vi "ICG_WD.vi"() -> ()   [LabVIEW 2020]
uses:
  <vilib>/Utility/file.llb/Read Delimited Spreadsheet (DBL).vi
  <vilib>/Analysis/NI_AALPro.lvlib
panel:
  out "SV 4":dbl
  out "SV 3":dbl
  out "SV 2":dbl
  out "SV":dbl
  out "SV":dbl
  out "Tlve 5":dbl
  out "interval7 2":dbl[](graph)
  out "location 5":dbl[](array[numeric])
  out "interval 7":dbl[](array[numeric])
  out "amplitude 5":dbl[](array[numeric])
  out "Amplitudes 5":dbl[](array[numeric])
  out "2nd Derivatives 5":dbl[](array[numeric])
  out "Locations 5":dbl[](array[numeric])
  out "max  4":dbl
  out "deltaZe(t)4 2":dbl[](graph)
  out "ICG array 5":dbl[](array[numeric])
  in  "file path (dialog if empty) 5":path
  out "Tlve 4":dbl
  out "interval7":dbl[](graph)
  out "location 4":dbl[](array[numeric])
  out "interval 6":dbl[](array[numeric])
  out "amplitude 4":dbl[](array[numeric])
  out "Amplitudes 4":dbl[](array[numeric])
  out "2nd Derivatives 4":dbl[](array[numeric])
  out "Locations 4":dbl[](array[numeric])
  out "max  3":dbl
  out "deltaZe(t)4":dbl[](graph)
  out "ICG array 4":dbl[](array[numeric])
  in  "file path (dialog if empty) 4":path
  out "Tlve 3":dbl
  out "interval 5":dbl[](graph)
  out "location 3":dbl[](array[numeric])
  out "interval 4":dbl[](array[numeric])
  out "amplitude 3":dbl[](array[numeric])
  out "Amplitudes 3":dbl[](array[numeric])
  out "2nd Derivatives 3":dbl[](array[numeric])
  out "Locations 3":dbl[](array[numeric])
  out "max  2":dbl
  out "deltaZe(t) 3":dbl[](graph)
  out "ICG array 3":dbl[](array[numeric])
  in  "file path (dialog if empty) 3":path
  out "Tlve 2":dbl
  out "interval 3":dbl[](graph)
  out "location 2":dbl[](array[numeric])
  out "interval 2":dbl[](array[numeric])
  out "amplitude 2":dbl[](array[numeric])
  out "Amplitudes 2":dbl[](array[numeric])
  out "2nd Derivatives 2":dbl[](array[numeric])
  out "Locations 2":dbl[](array[numeric])
  out "max  2":dbl
  out "deltaZe(t) 2":dbl[](graph)
  out "ICG":dbl[](array[numeric])
  in  "file path (dialog if empty) 2":path
  out "Tlve":dbl
  out "interval":dbl[](graph)
  out "location":dbl[](array[numeric])
  out "interval":dbl[](array[numeric])
  out "amplitude":dbl[](array[numeric])
  out "Amplitudes":dbl[](array[numeric])
  out "2nd Derivatives":dbl[](array[numeric])
  out "Locations":dbl[](array[numeric])
  out "max":dbl
  out "deltaZe(t)":dbl[](graph)
  out "ICG":dbl[](array[numeric])
  in  "file path (dialog if empty)":path
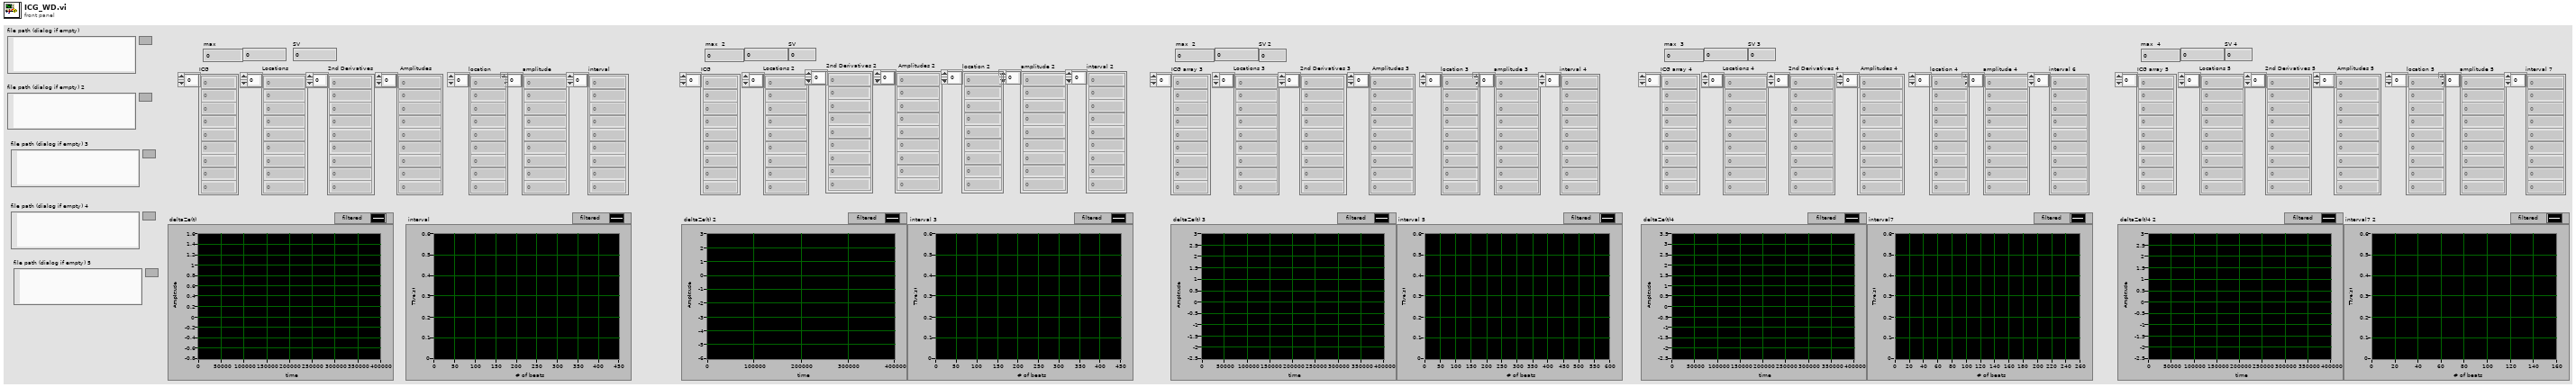
[diagram p1: front panel]
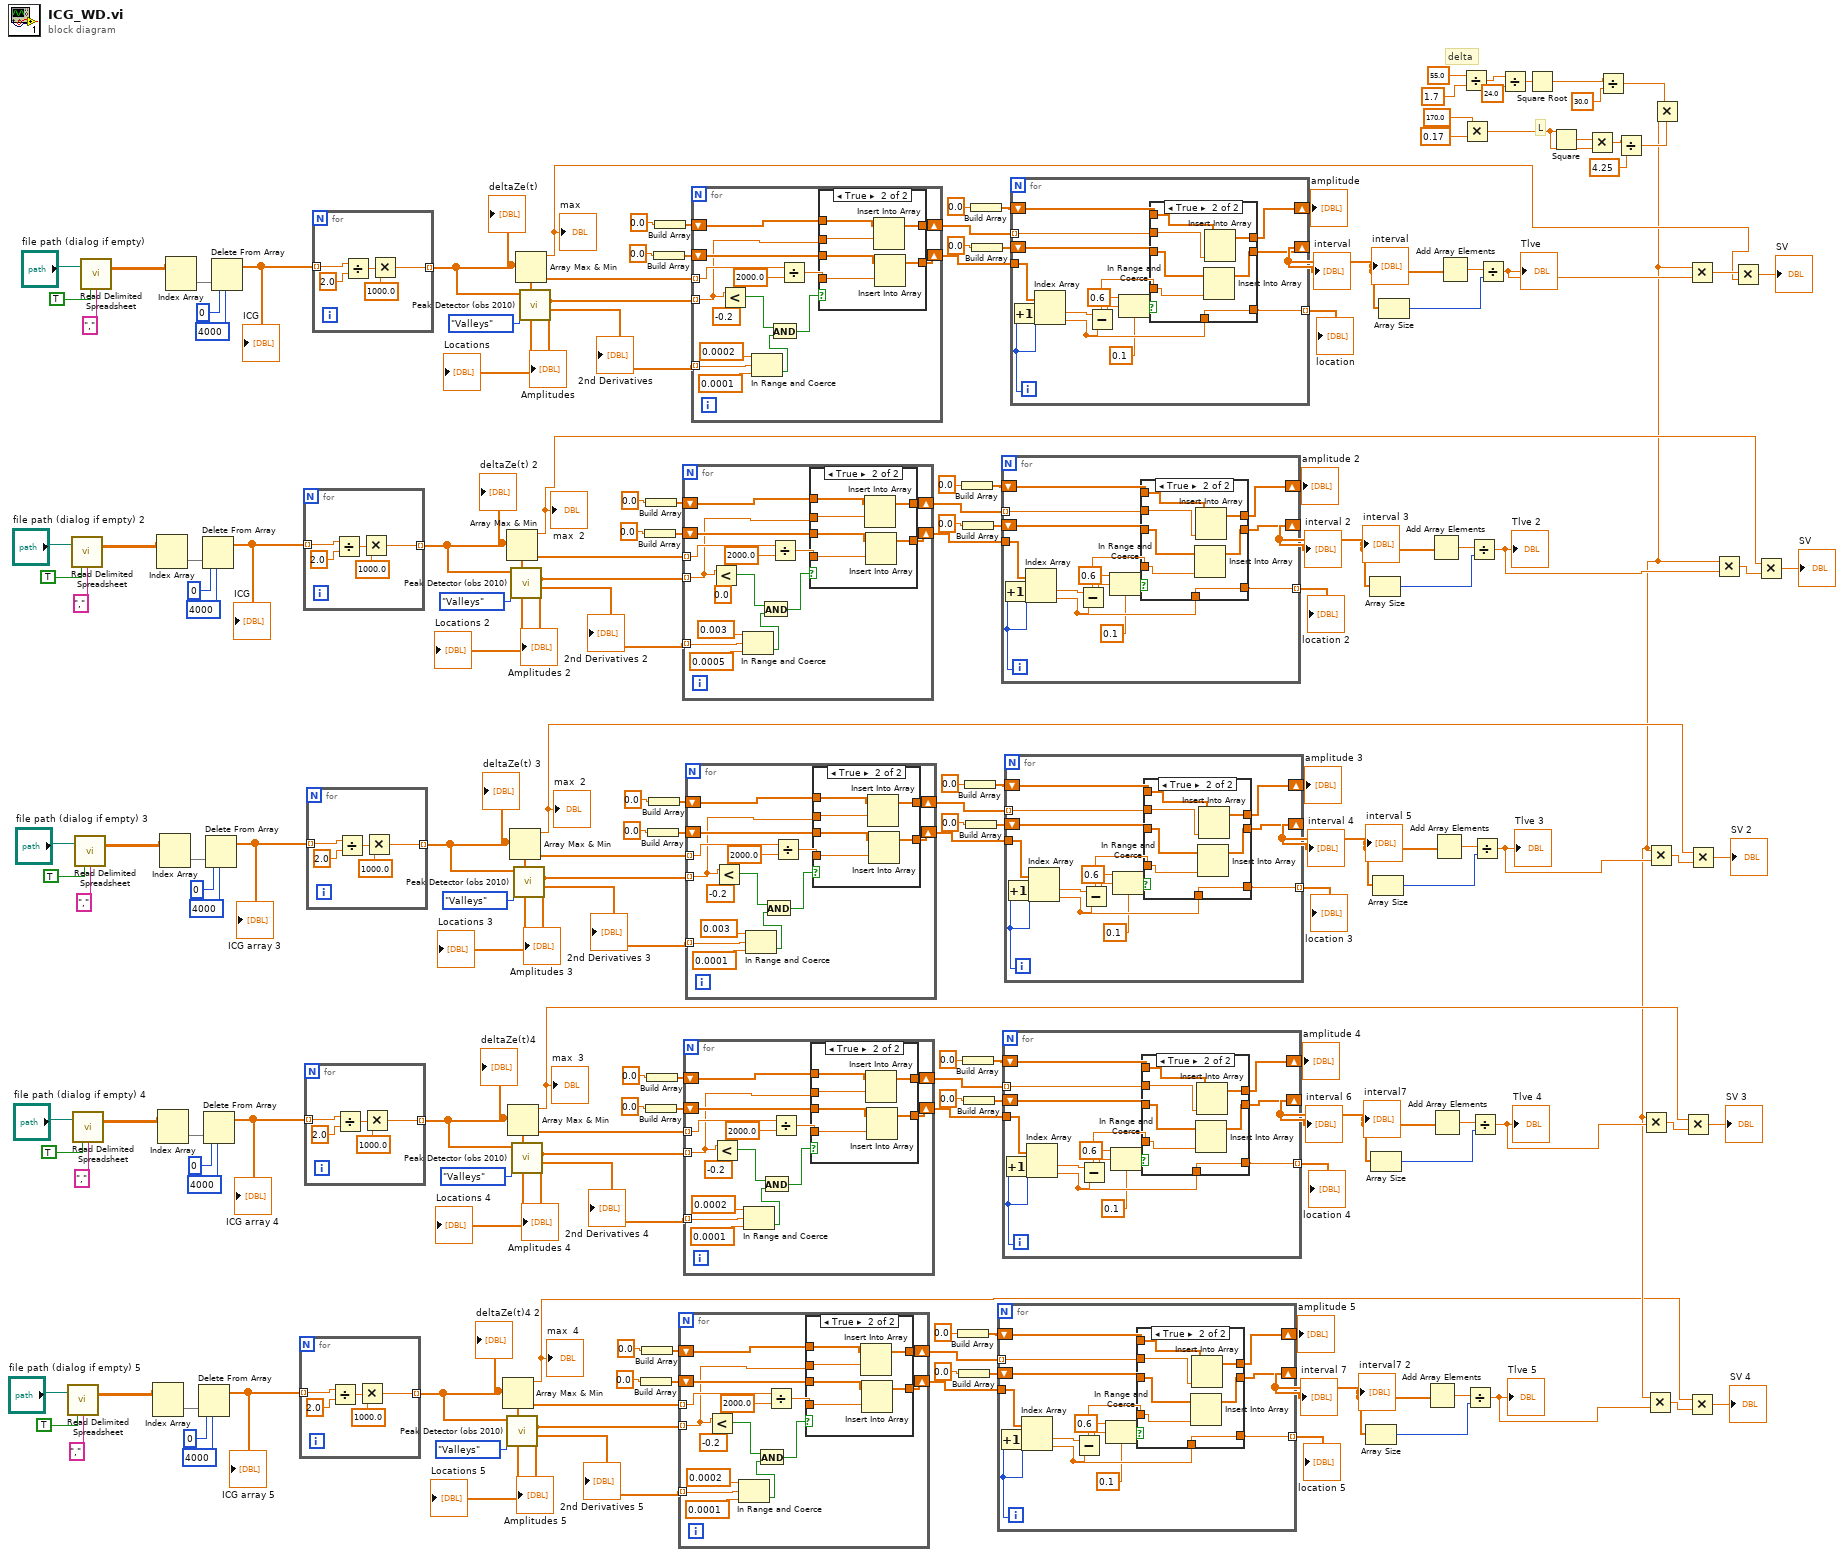
[diagram p0: block diagram]
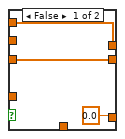
[diagram p2: hidden frame]
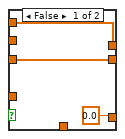
[diagram p4: hidden frame]
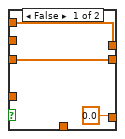
[diagram p6: hidden frame]
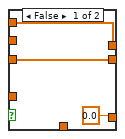
[diagram p8: hidden frame]
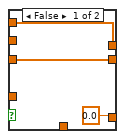
[diagram p10: hidden frame]
diagram:
  # "L"
  # "delta"
  n1 = call-poly <vilib>:"Read Delimited Spreadsheet.vi"("file path (dialog if empty)"="file path (dialog if empty) 5", "transpose? (F)"=TRUE, "delimiter (\\t)"="," ("delimiter (\\t)")) -> ("all rows"=w61:dbl[][])  [unwired: 7 in, 5 out]
  n2 = call-poly <vilib>:"Read Delimited Spreadsheet.vi"("file path (dialog if empty)"="file path (dialog if empty) 2", "transpose? (F)"=TRUE, "delimiter (\\t)"="," ("delimiter (\\t)")) -> ("all rows"=w145:dbl[][])  [unwired: 7 in, 5 out]
  n3 = call-poly <vilib>:"Read Delimited Spreadsheet.vi"("file path (dialog if empty)"="file path (dialog if empty) 4", "transpose? (F)"=TRUE, "delimiter (\\t)"="," ("delimiter (\\t)")) -> ("all rows"=w89:dbl[][])  [unwired: 7 in, 5 out]
  n4 = call-poly <vilib>:"Read Delimited Spreadsheet.vi"("file path (dialog if empty)"="file path (dialog if empty) 3", "transpose? (F)"=TRUE, "delimiter (\\t)"="," ("delimiter (\\t)")) -> ("all rows"=w117:dbl[][])  [unwired: 7 in, 5 out]
  n5 = call-poly <vilib>:"Read Delimited Spreadsheet.vi"("file path (dialog if empty)"="file path (dialog if empty)", "transpose? (F)"=TRUE, "delimiter (\\t)"="," ("delimiter (\\t)")) -> ("all rows"=w173:dbl[][])  [unwired: 7 in, 5 out]
  n6 = Index Array(array=w61) -> (element=w60:dbl[])  [unwired: 2 in]
  n7 = Index Array(array=w145) -> (element=w144:dbl[])  [unwired: 2 in]
  n8 = Index Array(array=w89) -> (element=w88:dbl[])  [unwired: 2 in]
  n9 = Index Array(array=w117) -> (element=w116:dbl[])  [unwired: 2 in]
  n10 = Index Array(array=w173) -> (element=w172:dbl[])  [unwired: 2 in]
  n11 = Delete From Array(array=w60, length=4000, index=0) -> (array with subset deleted=w57:dbl[])  [unwired: 1 out]
  "ICG array 5" <- w57
  n12 = Delete From Array(array=w144, length=4000, index=0) -> (array with subset deleted=w141:dbl[])  [unwired: 1 out]
  "ICG" <- w141
  n13 = Delete From Array(array=w88, length=4000, index=0) -> (array with subset deleted=w85:dbl[])  [unwired: 1 out]
  "ICG array 4" <- w85
  n14 = Delete From Array(array=w116, length=4000, index=0) -> (array with subset deleted=w113:dbl[])  [unwired: 1 out]
  "ICG array 3" <- w113
  n15 = Delete From Array(array=w172, length=4000, index=0) -> (array with subset deleted=w169:dbl[])  [unwired: 1 out]
  "ICG" <- w169
  n16 = for {
    tunnel: w57 -> [w181] mode=indexing
    tunnel: [w177] -> w53 mode=indexing
    n17 = Divide(x=w181, y=2.0) -> (x/y=w179:dbl)
    n18 = Multiply(x=w179, y=1000.0) -> (x*y=w177:dbl)
  }
  "deltaZe(t)4 2" <- w53
  n19 = for {
    tunnel: w141 -> [w186] mode=indexing
    tunnel: [w182] -> w137 mode=indexing
    n20 = Divide(x=w186, y=2.0) -> (x/y=w184:dbl)
    n21 = Multiply(x=w184, y=1000.0) -> (x*y=w182:dbl)
  }
  "deltaZe(t) 2" <- w137
  n22 = for {
    tunnel: w85 -> [w191] mode=indexing
    tunnel: [w187] -> w81 mode=indexing
    n23 = Divide(x=w191, y=2.0) -> (x/y=w189:dbl)
    n24 = Multiply(x=w189, y=1000.0) -> (x*y=w187:dbl)
  }
  "deltaZe(t)4" <- w81
  n25 = for {
    tunnel: w113 -> [w196] mode=indexing
    tunnel: [w192] -> w109 mode=indexing
    n26 = Divide(x=w196, y=2.0) -> (x/y=w194:dbl)
    n27 = Multiply(x=w194, y=1000.0) -> (x*y=w192:dbl)
  }
  "deltaZe(t) 3" <- w109
  n28 = for {
    tunnel: w169 -> [w201] mode=indexing
    tunnel: [w197] -> w165 mode=indexing
    n29 = Divide(x=w201, y=2.0) -> (x/y=w199:dbl)
    n30 = Multiply(x=w199, y=1000.0) -> (x*y=w197:dbl)
  }
  "deltaZe(t)" <- w165
  n31 = Array Max & Min(array=w53) -> (max value=w1:dbl)  [unwired: 3 out]
  "max  4" <- w1
  n32 = Array Max & Min(array=w137) -> (max value=w16:dbl)  [unwired: 3 out]
  "max  2" <- w16
  n33 = call <vilib>:"Peak Detector (obs 2010).vi"("peaks/valleys"=enum32{"Peaks", "Valleys"}."Valleys", "X"=w53) -> ("2nd Derivatives"=w51:dbl[], "Amplitudes"=w52:dbl[], "Locations"=w48:dbl[])  [unwired: 5 in, 2 out]
  "Locations 5" <- w48
  "2nd Derivatives 5" <- w51
  "Amplitudes 5" <- w52
  n34 = Array Max & Min(array=w81) -> (max value=w6:dbl)  [unwired: 3 out]
  "max  3" <- w6
  n35 = Array Max & Min(array=w109) -> (max value=w10:dbl)  [unwired: 3 out]
  "max  2" <- w10
  n36 = call <vilib>:"Peak Detector (obs 2010).vi"("peaks/valleys"=enum32{"Peaks", "Valleys"}."Valleys", "X"=w137) -> ("2nd Derivatives"=w135:dbl[], "Amplitudes"=w136:dbl[], "Locations"=w132:dbl[])  [unwired: 5 in, 2 out]
  "Locations 2" <- w132
  "2nd Derivatives 2" <- w135
  "Amplitudes 2" <- w136
  n37 = call <vilib>:"Peak Detector (obs 2010).vi"("peaks/valleys"=enum32{"Peaks", "Valleys"}."Valleys", "X"=w81) -> ("2nd Derivatives"=w79:dbl[], "Amplitudes"=w80:dbl[], "Locations"=w76:dbl[])  [unwired: 5 in, 2 out]
  "Locations 4" <- w76
  "2nd Derivatives 4" <- w79
  "Amplitudes 4" <- w80
  n38 = call <vilib>:"Peak Detector (obs 2010).vi"("peaks/valleys"=enum32{"Peaks", "Valleys"}."Valleys", "X"=w109) -> ("2nd Derivatives"=w107:dbl[], "Amplitudes"=w108:dbl[], "Locations"=w104:dbl[])  [unwired: 5 in, 2 out]
  "Locations 3" <- w104
  "2nd Derivatives 3" <- w107
  "Amplitudes 3" <- w108
  n39 = Array Max & Min(array=w165) -> (max value=w18:dbl)  [unwired: 3 out]
  "max" <- w18
  n40 = call <vilib>:"Peak Detector (obs 2010).vi"("peaks/valleys"=enum32{"Peaks", "Valleys"}."Valleys", "X"=w165) -> ("2nd Derivatives"=w163:dbl[], "Amplitudes"=w164:dbl[], "Locations"=w160:dbl[])  [unwired: 5 in, 2 out]
  "Locations" <- w160
  "2nd Derivatives" <- w163
  "Amplitudes" <- w164
  n41 = Build Array(0.0 ("array")) -> (w49:dbl[])
  n42 = Build Array(0.0 ("array")) -> (w54:dbl[])
  n43 = Build Array(0.0 ("array")) -> (w133:dbl[])
  n44 = Build Array(0.0 ("array")) -> (w138:dbl[])
  n45 = Build Array(0.0 ("array")) -> (w77:dbl[])
  n46 = Build Array(0.0 ("array")) -> (w82:dbl[])
  n47 = Build Array(0.0 ("array")) -> (w105:dbl[])
  n48 = Build Array(0.0 ("array")) -> (w110:dbl[])
  n49 = Build Array(0.0 ("array")) -> (w161:dbl[])
  n50 = Build Array(0.0 ("array")) -> (w166:dbl[])
  n51 = for {
    tunnel: w52 -> [w202] mode=indexing
    shift-right: [w214] -> w47
    shift-left: w54 -> [w215]
    tunnel: w51 -> [w209] mode=indexing
    shift-right: [w207] -> w46
    shift-left: w49 -> [w208]
    tunnel: w48 -> [w205] mode=indexing
    n52 = Less?(x=w202, y=-0.2) -> (x < y?=w211:bool)
    n53 = In Range and Coerce(upper limit=0.0002, x=w209, lower limit=0.0001) -> (In Range?=w206:bool)  [unwired: 1 out]
    n54 = And(x=w211, y=w206) -> (x .and. y?=w210:bool)
    n55 = Divide(x=w205, y=2000.0) -> (x/y=w203:dbl)
    n56 = case shown="True" w210 {
      tunnel: w215 -> [w218 w224]
      tunnel: [w218 w223] -> w214
      tunnel: w202 -> [_ w222]
      tunnel: w208 -> [w217 w221]
      tunnel: [w217 w220] -> w207
      tunnel: w203 -> [_ w219]
      frame False {
      }
      frame True {
        n57 = Insert Into Array(array=w224, new element=w222) -> (w223:dbl[])  [unwired: 1 in]
        n58 = Insert Into Array(array=w221, new element=w219) -> (w220:dbl[])  [unwired: 1 in]
      }
    }
  }
  n59 = for {
    tunnel: w136 -> [w225] mode=indexing
    shift-right: [w237] -> w131
    shift-left: w138 -> [w238]
    tunnel: w135 -> [w232] mode=indexing
    shift-right: [w230] -> w130
    shift-left: w133 -> [w231]
    tunnel: w132 -> [w228] mode=indexing
    n60 = Less?(x=w225, y=0.0) -> (x < y?=w234:bool)
    n61 = In Range and Coerce(upper limit=0.003, x=w232, lower limit=0.0005) -> (In Range?=w229:bool)  [unwired: 1 out]
    n62 = And(x=w234, y=w229) -> (x .and. y?=w233:bool)
    n63 = Divide(x=w228, y=2000.0) -> (x/y=w226:dbl)
    n64 = case shown="True" w233 {
      tunnel: w238 -> [w241 w247]
      tunnel: [w241 w246] -> w237
      tunnel: w225 -> [_ w245]
      tunnel: w231 -> [w240 w244]
      tunnel: [w240 w243] -> w230
      tunnel: w226 -> [_ w242]
      frame False {
      }
      frame True {
        n65 = Insert Into Array(array=w247, new element=w245) -> (w246:dbl[])  [unwired: 1 in]
        n66 = Insert Into Array(array=w244, new element=w242) -> (w243:dbl[])  [unwired: 1 in]
      }
    }
  }
  n67 = for {
    tunnel: w80 -> [w248] mode=indexing
    shift-right: [w260] -> w75
    shift-left: w82 -> [w261]
    tunnel: w79 -> [w255] mode=indexing
    shift-right: [w253] -> w74
    shift-left: w77 -> [w254]
    tunnel: w76 -> [w251] mode=indexing
    n68 = Less?(x=w248, y=-0.2) -> (x < y?=w257:bool)
    n69 = In Range and Coerce(upper limit=0.0002, x=w255, lower limit=0.0001) -> (In Range?=w252:bool)  [unwired: 1 out]
    n70 = And(x=w257, y=w252) -> (x .and. y?=w256:bool)
    n71 = Divide(x=w251, y=2000.0) -> (x/y=w249:dbl)
    n72 = case shown="True" w256 {
      tunnel: w261 -> [w264 w270]
      tunnel: [w264 w269] -> w260
      tunnel: w248 -> [_ w268]
      tunnel: w254 -> [w263 w267]
      tunnel: [w263 w266] -> w253
      tunnel: w249 -> [_ w265]
      frame False {
      }
      frame True {
        n73 = Insert Into Array(array=w270, new element=w268) -> (w269:dbl[])  [unwired: 1 in]
        n74 = Insert Into Array(array=w267, new element=w265) -> (w266:dbl[])  [unwired: 1 in]
      }
    }
  }
  n75 = for {
    tunnel: w108 -> [w271] mode=indexing
    shift-right: [w283] -> w103
    shift-left: w110 -> [w284]
    tunnel: w107 -> [w278] mode=indexing
    shift-right: [w276] -> w102
    shift-left: w105 -> [w277]
    tunnel: w104 -> [w274] mode=indexing
    n76 = Less?(x=w271, y=-0.2) -> (x < y?=w280:bool)
    n77 = In Range and Coerce(upper limit=0.003, x=w278, lower limit=0.0001) -> (In Range?=w275:bool)  [unwired: 1 out]
    n78 = And(x=w280, y=w275) -> (x .and. y?=w279:bool)
    n79 = Divide(x=w274, y=2000.0) -> (x/y=w272:dbl)
    n80 = case shown="True" w279 {
      tunnel: w284 -> [w287 w293]
      tunnel: [w287 w292] -> w283
      tunnel: w271 -> [_ w291]
      tunnel: w277 -> [w286 w290]
      tunnel: [w286 w289] -> w276
      tunnel: w272 -> [_ w288]
      frame False {
      }
      frame True {
        n81 = Insert Into Array(array=w293, new element=w291) -> (w292:dbl[])  [unwired: 1 in]
        n82 = Insert Into Array(array=w290, new element=w288) -> (w289:dbl[])  [unwired: 1 in]
      }
    }
  }
  n83 = for {
    tunnel: w164 -> [w294] mode=indexing
    shift-right: [w306] -> w159
    shift-left: w166 -> [w307]
    tunnel: w163 -> [w301] mode=indexing
    shift-right: [w299] -> w158
    shift-left: w161 -> [w300]
    tunnel: w160 -> [w297] mode=indexing
    n84 = Less?(x=w294, y=-0.2) -> (x < y?=w303:bool)
    n85 = In Range and Coerce(upper limit=0.0002, x=w301, lower limit=0.0001) -> (In Range?=w298:bool)  [unwired: 1 out]
    n86 = And(x=w303, y=w298) -> (x .and. y?=w302:bool)
    n87 = Divide(x=w297, y=2000.0) -> (x/y=w295:dbl)
    n88 = case shown="True" w302 {
      tunnel: w307 -> [w310 w316]
      tunnel: [w310 w315] -> w306
      tunnel: w294 -> [_ w314]
      tunnel: w300 -> [w309 w313]
      tunnel: [w309 w312] -> w299
      tunnel: w295 -> [_ w311]
      frame False {
      }
      frame True {
        n89 = Insert Into Array(array=w316, new element=w314) -> (w315:dbl[])  [unwired: 1 in]
        n90 = Insert Into Array(array=w313, new element=w311) -> (w312:dbl[])  [unwired: 1 in]
      }
    }
  }
  n91 = Build Array(0.0 ("array")) -> (w43:dbl[])
  n92 = Build Array(0.0 ("array")) -> (w44:dbl[])
  n93 = Build Array(0.0 ("array")) -> (w127:dbl[])
  n94 = Build Array(0.0 ("array")) -> (w128:dbl[])
  n95 = Build Array(0.0 ("array")) -> (w71:dbl[])
  n96 = Build Array(0.0 ("array")) -> (w72:dbl[])
  n97 = Build Array(0.0 ("array")) -> (w99:dbl[])
  n98 = Build Array(0.0 ("array")) -> (w100:dbl[])
  n99 = Build Array(0.0 ("array")) -> (w155:dbl[])
  n100 = Build Array(0.0 ("array")) -> (w156:dbl[])
  n101 = for {
    tunnel: w46 -> [w329]
    shift-right: [w325] -> w39
    shift-left: w44 -> [w326]
    tunnel: w47 -> [w321] mode=indexing
    shift-right: [w331] -> w41
    shift-left: w43 -> [w324]
    tunnel: [w322] -> w40 mode=indexing
    i -> [w328]
    n102 = Increment(x=w328) -> (x+1=w330:i32)
    n103 = Index Array(array=w329, index #1=w330, index #2=w328) -> (element #1=w327:dbl, element #2=w323:dbl)
    n104 = Subtract(x=w327, y=w323) -> (x-y=w317:dbl)
    n105 = In Range and Coerce(upper limit=0.6, x=w317, lower limit=0.1 ("y")) -> (In Range?=w320:bool)  [unwired: 1 out]
    n106 = case shown="True" w320 {
      tunnel: w321 -> [_ w337]
      tunnel: [w333 w341] -> w331
      tunnel: w326 -> [w334 w340]
      tunnel: [w334 w339] -> w325
      tunnel: w324 -> [w333 w338]
      tunnel: w317 -> [_ w336]
      tunnel: w323 -> [_ w335]
      tunnel: [0.0 ("array") w335] -> w322
      frame False {
      }
      frame True {
        n107 = Insert Into Array(array=w340, new element=w336) -> (w339:dbl[])  [unwired: 1 in]
        n108 = Insert Into Array(array=w338, new element=w337) -> (w341:dbl[])  [unwired: 1 in]
      }
    }
  }
  "amplitude 5" <- w41
  "interval 7" <- w39
  "location 5" <- w40
  "interval7 2" <- w39
  n109 = for {
    tunnel: w130 -> [w354]
    shift-right: [w350] -> w123
    shift-left: w128 -> [w351]
    tunnel: w131 -> [w346] mode=indexing
    shift-right: [w356] -> w125
    shift-left: w127 -> [w349]
    tunnel: [w347] -> w124 mode=indexing
    i -> [w353]
    n110 = Increment(x=w353) -> (x+1=w355:i32)
    n111 = Index Array(array=w354, index #1=w355, index #2=w353) -> (element #1=w352:dbl, element #2=w348:dbl)
    n112 = Subtract(x=w352, y=w348) -> (x-y=w342:dbl)
    n113 = In Range and Coerce(upper limit=0.6, x=w342, lower limit=0.1 ("y")) -> (In Range?=w345:bool)  [unwired: 1 out]
    n114 = case shown="True" w345 {
      tunnel: w346 -> [_ w362]
      tunnel: [w358 w366] -> w356
      tunnel: w351 -> [w359 w365]
      tunnel: [w359 w364] -> w350
      tunnel: w349 -> [w358 w363]
      tunnel: w342 -> [_ w361]
      tunnel: w348 -> [_ w360]
      tunnel: [0.0 ("array") w360] -> w347
      frame False {
      }
      frame True {
        n115 = Insert Into Array(array=w365, new element=w361) -> (w364:dbl[])  [unwired: 1 in]
        n116 = Insert Into Array(array=w363, new element=w362) -> (w366:dbl[])  [unwired: 1 in]
      }
    }
  }
  "amplitude 2" <- w125
  "interval 2" <- w123
  "location 2" <- w124
  "interval 3" <- w123
  n117 = for {
    tunnel: w74 -> [w379]
    shift-right: [w375] -> w67
    shift-left: w72 -> [w376]
    tunnel: w75 -> [w371] mode=indexing
    shift-right: [w381] -> w69
    shift-left: w71 -> [w374]
    tunnel: [w372] -> w68 mode=indexing
    i -> [w378]
    n118 = Increment(x=w378) -> (x+1=w380:i32)
    n119 = Index Array(array=w379, index #1=w380, index #2=w378) -> (element #1=w377:dbl, element #2=w373:dbl)
    n120 = Subtract(x=w377, y=w373) -> (x-y=w367:dbl)
    n121 = In Range and Coerce(upper limit=0.6, x=w367, lower limit=0.1 ("y")) -> (In Range?=w370:bool)  [unwired: 1 out]
    n122 = case shown="True" w370 {
      tunnel: w371 -> [_ w387]
      tunnel: [w383 w391] -> w381
      tunnel: w376 -> [w384 w390]
      tunnel: [w384 w389] -> w375
      tunnel: w374 -> [w383 w388]
      tunnel: w367 -> [_ w386]
      tunnel: w373 -> [_ w385]
      tunnel: [0.0 ("array") w385] -> w372
      frame False {
      }
      frame True {
        n123 = Insert Into Array(array=w390, new element=w386) -> (w389:dbl[])  [unwired: 1 in]
        n124 = Insert Into Array(array=w388, new element=w387) -> (w391:dbl[])  [unwired: 1 in]
      }
    }
  }
  "amplitude 4" <- w69
  "interval 6" <- w67
  "location 4" <- w68
  "interval7" <- w67
  n125 = for {
    tunnel: w102 -> [w404]
    shift-right: [w400] -> w95
    shift-left: w100 -> [w401]
    tunnel: w103 -> [w396] mode=indexing
    shift-right: [w406] -> w97
    shift-left: w99 -> [w399]
    tunnel: [w397] -> w96 mode=indexing
    i -> [w403]
    n126 = Increment(x=w403) -> (x+1=w405:i32)
    n127 = Index Array(array=w404, index #1=w405, index #2=w403) -> (element #1=w402:dbl, element #2=w398:dbl)
    n128 = Subtract(x=w402, y=w398) -> (x-y=w392:dbl)
    n129 = In Range and Coerce(upper limit=0.6, x=w392, lower limit=0.1 ("y")) -> (In Range?=w395:bool)  [unwired: 1 out]
    n130 = case shown="True" w395 {
      tunnel: w396 -> [_ w412]
      tunnel: [w408 w416] -> w406
      tunnel: w401 -> [w409 w415]
      tunnel: [w409 w414] -> w400
      tunnel: w399 -> [w408 w413]
      tunnel: w392 -> [_ w411]
      tunnel: w398 -> [_ w410]
      tunnel: [0.0 ("array") w410] -> w397
      frame False {
      }
      frame True {
        n131 = Insert Into Array(array=w415, new element=w411) -> (w414:dbl[])  [unwired: 1 in]
        n132 = Insert Into Array(array=w413, new element=w412) -> (w416:dbl[])  [unwired: 1 in]
      }
    }
  }
  "amplitude 3" <- w97
  "interval 4" <- w95
  "location 3" <- w96
  "interval 5" <- w95
  n133 = for {
    tunnel: w158 -> [w429]
    shift-right: [w417] -> w151
    shift-left: w156 -> [w426]
    tunnel: w159 -> [w422] mode=indexing
    shift-right: [w431] -> w153
    shift-left: w155 -> [w425]
    tunnel: [w423] -> w152 mode=indexing
    i -> [w428]
    n134 = Increment(x=w428) -> (x+1=w430:i32)
    n135 = Index Array(array=w429, index #1=w430, index #2=w428) -> (element #1=w427:dbl, element #2=w424:dbl)
    n136 = Subtract(x=w427, y=w424) -> (x-y=w418:dbl)
    n137 = In Range and Coerce(upper limit=0.6, x=w418, lower limit=0.1 ("y")) -> (In Range?=w421:bool)  [unwired: 1 out]
    n138 = case shown="True" w421 {
      tunnel: w422 -> [_ w437]
      tunnel: [w433 w441] -> w431
      tunnel: w426 -> [w434 w440]
      tunnel: [w434 w439] -> w417
      tunnel: w425 -> [w433 w438]
      tunnel: w418 -> [_ w436]
      tunnel: w424 -> [_ w435]
      tunnel: [0.0 ("array") w435] -> w423
      frame False {
      }
      frame True {
        n139 = Insert Into Array(array=w440, new element=w436) -> (w439:dbl[])  [unwired: 1 in]
        n140 = Insert Into Array(array=w438, new element=w437) -> (w441:dbl[])  [unwired: 1 in]
      }
    }
  }
  "amplitude" <- w153
  "interval" <- w151
  "location" <- w152
  "interval" <- w151
  n141 = Array Size(array=w39) -> (size(s)=w37:i32)
  n142 = Array Size(array=w123) -> (size(s)=w121:i32)
  n143 = Array Size(array=w67) -> (size(s)=w65:i32)
  n144 = Array Size(array=w95) -> (size(s)=w93:i32)
  n145 = Array Size(array=w151) -> (size(s)=w149:i32)
  n146 = Add Array Elements(numeric array=w39) -> (sum=w38:dbl)
  n147 = Add Array Elements(numeric array=w123) -> (sum=w122:dbl)
  n148 = Add Array Elements(numeric array=w67) -> (sum=w66:dbl)
  n149 = Add Array Elements(numeric array=w95) -> (sum=w94:dbl)
  n150 = Add Array Elements(numeric array=w151) -> (sum=w150:dbl)
  n151 = Divide(x=55.0, y=1.7) -> (x/y=w24:dbl)
  n152 = Multiply(x=170.0, y=0.17) -> (x*y=w31:dbl)
  n153 = Divide(x=w38, y=w37) -> (x/y=w3:dbl)
  "Tlve 5" <- w3
  n154 = Divide(x=w122, y=w121) -> (x/y=w17:dbl)
  "Tlve 2" <- w17
  n155 = Divide(x=w66, y=w65) -> (x/y=w7:dbl)
  "Tlve 4" <- w7
  n156 = Divide(x=w94, y=w93) -> (x/y=w11:dbl)
  "Tlve 3" <- w11
  n157 = Divide(x=w150, y=w149) -> (x/y=w27:dbl)
  "Tlve" <- w27
  n158 = Divide(x=w24, y=24.0) -> (x/y=w22:dbl)
  n159 = Square Root(x=w22) -> (sqrt(x)=w20:dbl)
  n160 = Square(x=w31) -> (x^2=w32:dbl)
  n161 = Multiply(x=w32, y=w31) -> (x*y=w30:dbl)
  n162 = Divide(x=w20, y=30.0) -> (x/y=w29:dbl)
  n163 = Divide(x=w30, y=4.25) -> (x/y=w28:dbl)
  n164 = Multiply(x=w29, y=w28) -> (x*y=w2:dbl)
  n165 = Multiply(x=w2, y=w7) -> (x*y=w9:dbl)
  n166 = Multiply(x=w2, y=w3) -> (x*y=w5:dbl)
  n167 = Multiply(x=w2, y=w11) -> (x*y=w13:dbl)
  n168 = Multiply(x=w6, y=w9) -> (x*y=→"SV 3":dbl)
  n169 = Multiply(x=w2, y=w27) -> (x*y=w26:dbl)
  n170 = Multiply(x=w1, y=w5) -> (x*y=→"SV 4":dbl)
  n171 = Multiply(x=w10, y=w13) -> (x*y=→"SV 2":dbl)
  n172 = Multiply(x=w2, y=w17) -> (x*y=w15:dbl)
  n173 = Multiply(x=w26, y=w18) -> (x*y=→"SV":dbl)
  n174 = Multiply(x=w16, y=w15) -> (x*y=→"SV":dbl)
